vi "InternalStacking.vi"(7 "Cancel Internal Stacking":bool, 10 "Initialize Internal Stacking":bool) -> ()   [LabVIEW 2014]
uses:
  2015 Main Project/InternalStacking.ctl
  2015 Main Project/Robot Global Data.vi
panel:
  in  "Winch Sensor Position":dbl
  out "Winch Cims Setpoint":dbl
  out "Internal Stacking Plate (set)":dbl
  in  "Tote Num Get":dbl
  out "Tote Num Set":dbl
  out "State of Elevator":T1
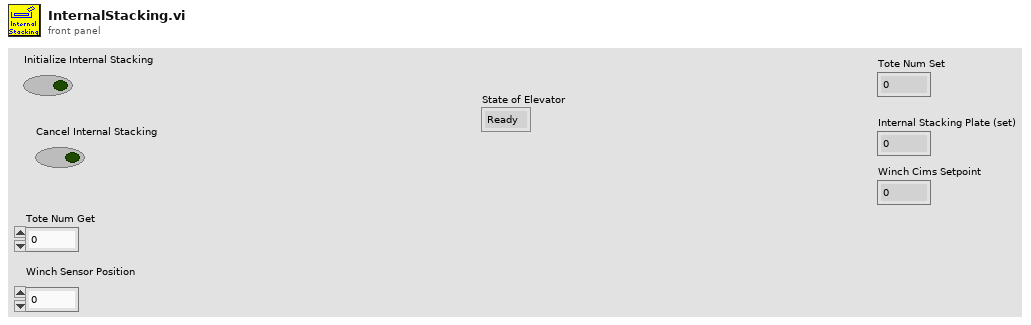
[diagram p1: front panel]
types:
  T1 = typedef "InternalStacking.ctl" = enum16{"Ready", "Extend Plate", "Lift Tote", "Wait For Seated Tote", "Release Tote", "Reset To Bottom Limit ", "Emergency Cancel"}
  T2 = typedef "WPI_ServoDeviceRef.ctl" = cluster{"DeviceStatus":errorcluster, "Controller":T3, "PWM Channel":T4, "DeadBand":T5}
  T3 = typedef "FPGA_TypedefDigitalModule.ctl" = enum16{"Controller 1"}
  T4 = typedef "FPGA_DIOPWMChannel.ctl" = enum8{"PWM 0", "PWM 1", "PWM 2", "PWM 3", "PWM 4", "PWM 5", "PWM 6", "PWM 7", "PWM 8", "PWM 9", "PWM MXP 0", "PWM MXP 1", "PWM MXP 2", "PWM MXP 3", "PWM MXP 4", "PWM MXP 5", "PWM MXP 6", "PWM MXP 7", "PWM MXP 8", "PWM MXP 9", "Invalid"}
  T5 = typedef "WPI_PWMDeadband.ctl" = cluster{"Name":string, "maxPositivePwm":i32, "minPositivePwm":i32, "centerPwm":i32, "maxNegativePwm":i32, "minNegativePwm":i32, "angularRange":u16}
  T6 = typedef "WPI_MotorControlDeviceRef.ctl" = cluster{"DeviceStatus":errorcluster, "Type":T7, "PWM":cluster{"Controller":T3, "PWM Channel":T4, "DeadBand":T5}, "CAN":cluster{"Device Number":u8, "Control Mode":T8, "Semaphore":T9, "Max Vout":dbl, "TalonSRX Control Mode":T10}, "Invert":bool, "TransformRef":T11, "InvTransformRef":T11}
  T7 = typedef "WPI_MotorControlType.ctl" = enum16{"PWM", "CAN", "CANTalonSRX"}
  T8 = typedef "WPI_CANJaguar_ControlMode.ctl" = enum8{"Percent VBus", "Current", "Speed", "Position", "Voltage"}
  T9 = typedef "Semaphore RefNum" = refnum<k1>
  T10 = typedef "WPI_CANTalonSRX_APIControlMode.ctl" = enum8{"Percent VBus", "Speed", "Position", "Slave", "Unchanged / Invalid"}
  T11 = typedef "WPI_PWMTransform_ConPane.ctl" = refnum<vi>
  T12 = typedef "WPI_CANTalonSRX_GlobalStatus.ctl" = cluster{"Applied Throttle":dbl, "Module Enabled":bool, "CAN Error":errorcluster, "Closed Loop Error":dbl, "Forward Limit Switch Closed":bool, "Reverse Limit Switch Closed":bool, "Sensor Position":dbl, "Sensor Velocity":dbl, "Current":dbl, "Sticky Fault - Over Temp":bool, "Sticky Fault - Under Voltage":bool, "Sticky Fault - Forward Limit":bool, "Sticky Fault - Reverse Limit":bool, "Sticky Fault - Forward Soft Limit":bool, "Sticky Fault - Reverse Soft Limit":bool, "Brake is Enabled":bool, "Encoder Position":dbl, "Encoder Velocity":dbl, "Encoder Index Count":dbl, "Encoder A Pin State":bool, "Encoder B Pin State":bool, "Encoder Index Pin State":bool, "Analog In":dbl, "Analog In Velocity":dbl, "Temperature (C)":dbl, "Battery Voltage":dbl}
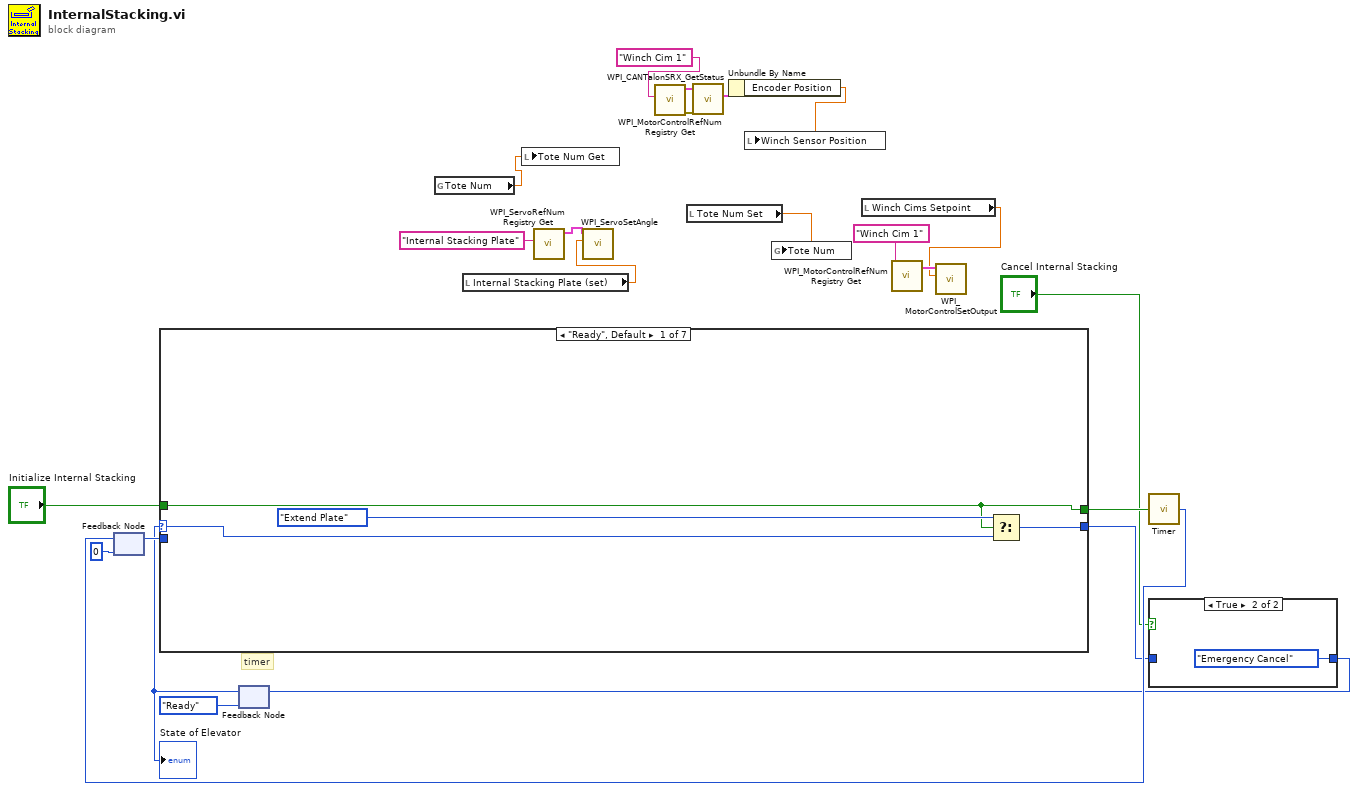
[diagram p0: block diagram]
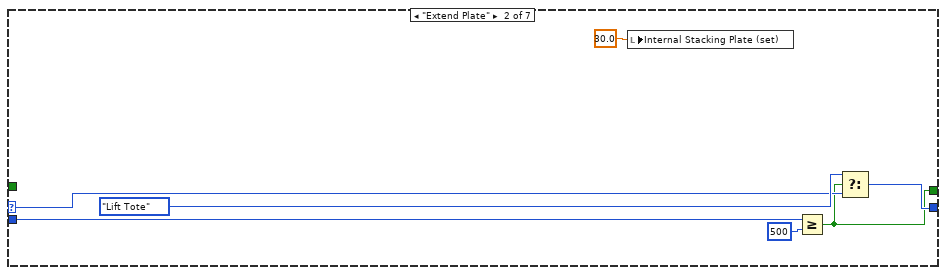
[diagram p3: hidden frame]
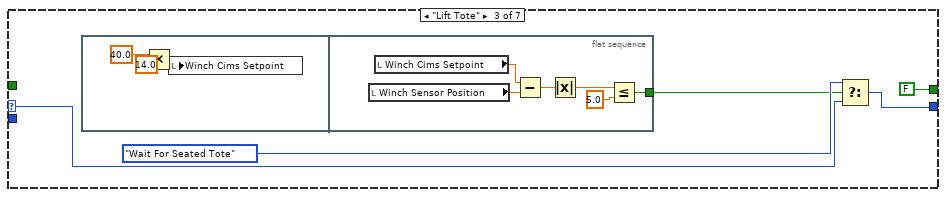
[diagram p4: hidden frame]
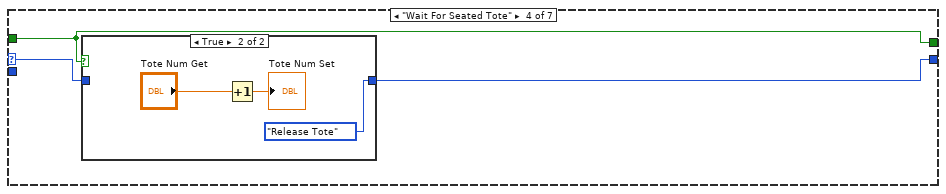
[diagram p5: hidden frame]
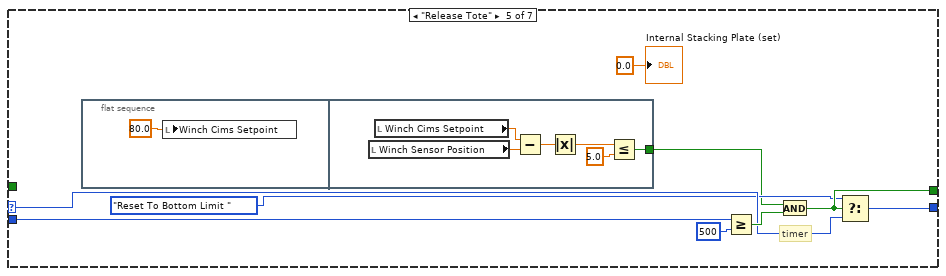
[diagram p7: hidden frame]
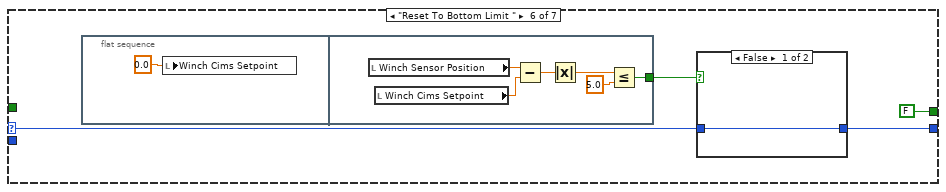
[diagram p8: hidden frame]
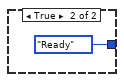
[diagram p9: hidden frame]
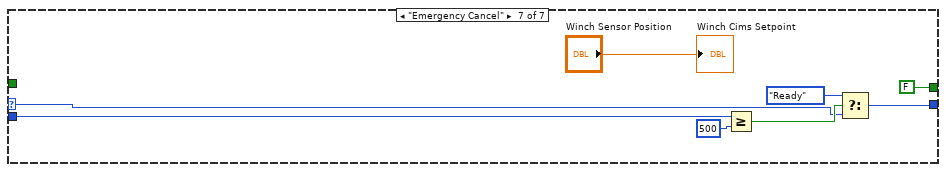
[diagram p10: hidden frame]
diagram:
  # "timer"
  n1 = feedback #1(u64 0 ("Time elapsed")) -> (w20:u64)
  n2 = feedback #2(InternalStacking."Ready" ("State of Elevator")) -> (w14:T1)
  "State of Elevator" <- w14
  n3 = case shown="\"Ready\", Default" w14 {
    selector: w14 -> [w26 w33 w38 w49 w60 w74 w88]
    tunnel: "Initialize Internal Stacking" -> [w24 _ _ w51 _ _ _]
    tunnel: [w25 w32 w37 w50 w58 w75 w87] -> w17
    tunnel: [w24 w29 FALSE ("Initialize Internal Stacking") w51 w61 FALSE ("Initialize Internal Stacking") FALSE] -> w22
    tunnel: w20 -> [_ w31 _ _ w64 _ w86]
    frame "Ready", Default {
      n4 = Select(t=InternalStacking."Extend Plate" ("State of Elevator"), s=w24, f=w26) -> (s? t:f=w25:T1)
    }
    frame "Extend Plate" {
      n5 = local write "Internal Stacking Plate (set)"(30.0 ("Internal Stacking Plate (set)")) -> ()
      n6 = Greater Or Equal?(x=w31, y=500) -> (x >= y?=w29:bool)
      n7 = Select(t=InternalStacking."Lift Tote" ("State of Elevator"), s=w29, f=w33) -> (s? t:f=w32:T1)
    }
    frame "Lift Tote" {
      n8 = flat-sequence {
        tunnel: [w43] -> w36
        frame #0 {
          n9 = Multiply(x=40.0, y=14.0 ("Ejector Motor Set")) -> (x*y=w41:dbl)
          n10 = local write "Winch Cims Setpoint"(w41) -> ()
        }
        frame #1 {
          n11 = local read "Winch Sensor Position"() -> (w48:dbl)
          n12 = local read "Winch Cims Setpoint"() -> (w47:dbl)
          n13 = Subtract(x=w47, y=w48) -> (x-y=w46:dbl)
          n14 = Absolute Value(x=w46) -> (abs(x)=w45:dbl)
          n15 = Less Or Equal?(x=w45, y=5.0) -> (x <= y?=w43:bool)
        }
      }
      n16 = Select(t=InternalStacking."Wait For Seated Tote" ("State of Elevator"), s=w36, f=w38) -> (s? t:f=w37:T1)
    }
    frame "Wait For Seated Tote" {
      n17 = case shown="True" w51 {
        tunnel: [w52 InternalStacking."Release Tote" ("State of Elevator")] -> w50
        tunnel: w49 -> [w52 _]
        frame False {
        }
        frame True {
          n18 = Increment(x="Tote Num Get") -> (x+1=→"Tote Num Set":dbl)
        }
      }
    }
    frame "Release Tote" {
      # "timer"
      n19 = flat-sequence {
        tunnel: [w66] -> w57
        frame #0 {
          n20 = local write "Winch Cims Setpoint"(80.0 ("Ejector Motor Set")) -> ()
        }
        frame #1 {
          n21 = local read "Winch Sensor Position"() -> (w71:dbl)
          n22 = local read "Winch Cims Setpoint"() -> (w70:dbl)
          n23 = Subtract(x=w70, y=w71) -> (x-y=w69:dbl)
          n24 = Absolute Value(x=w69) -> (abs(x)=w68:dbl)
          n25 = Less Or Equal?(x=w68, y=5.0) -> (x <= y?=w66:bool)
        }
      }
      n26 = Greater Or Equal?(x=w64, y=u64 500) -> (x >= y?=w62:bool)
      n27 = And(x=w57, y=w62) -> (x .and. y?=w61:bool)
      n28 = Select(t=InternalStacking."Reset To Bottom Limit " ("State of Elevator"), s=w61, f=w60) -> (s? t:f=w58:T1)
      "Internal Stacking Plate (set)" <- 0.0 ("Internal Stacking Plate (set)")
    }
    frame "Reset To Bottom Limit " {
      n29 = flat-sequence {
        tunnel: [w77] -> w73
        frame #0 {
          n30 = local write "Winch Cims Setpoint"(0.0 ("Ejector Motor Set")) -> ()
        }
        frame #1 {
          n31 = local read "Winch Sensor Position"() -> (w81:dbl)
          n32 = local read "Winch Cims Setpoint"() -> (w82:dbl)
          n33 = Subtract(x=w81, y=w82) -> (x-y=w80:dbl)
          n34 = Absolute Value(x=w80) -> (abs(x)=w79:dbl)
          n35 = Less Or Equal?(x=w79, y=5.0) -> (x <= y?=w77:bool)
        }
      }
      n36 = case shown="False" w73 {
        tunnel: [w83 InternalStacking."Ready" ("State of Elevator")] -> w75
        tunnel: w74 -> [w83 _]
        frame False {
        }
        frame True {
        }
      }
    }
    frame "Emergency Cancel" {
      n37 = Greater Or Equal?(x=w86, y=u64 500) -> (x >= y?=w90:bool)
      n38 = Select(t=InternalStacking."Ready" ("State of Elevator"), s=w90, f=w88) -> (s? t:f=w87:T1)
      "Winch Cims Setpoint" <- "Winch Sensor Position"
    }
  }
  n39 = global read "Robot Global Data.vi" "Tote Num"() -> (w13:dbl)
  n40 = local read "Internal Stacking Plate (set)"() -> (w10:dbl)
  n41 = local write "Tote Num Get"(w13) -> ()
  n42 = call <vilib>:"WPI_ServoRefNum Registry Get.vi"("refnum name"="Internal Stacking Plate") -> ("ServoDeviceRef"=w9:T2)  [unwired: 9 in, 1 out]
  n43 = call <vilib>:"WPI_ServoSetAngle.vi"("Angle"=w10, "ServoDeviceRef"=w9) -> ()  [unwired: 8 in, 2 out]
  n44 = call <vilib>:"WPI_MotorControlRefNum Registry Get.vi"("refnum name"="Winch Cim 1") -> ("error out"=w6:errorcluster, "MotorControlDevRef"=w7:T6)  [unwired: 9 in]
  n45 = local read "Tote Num Set"() -> (w12:dbl)
  n46 = call <vilib>:"WPI_CANTalonSRX_GetStatus.vi"("error in (no error)"=w6, "CAN Talon SRX Ref"=w7) -> ("Talon SRX Status"=w8:T12)  [unwired: 7 in, 2 out]
  n47 = Unbundle By Name(w8) -> ("Encoder Position"=w5:dbl)
  n48 = local write "Winch Sensor Position"(w5) -> ()
  n49 = global write "Robot Global Data.vi" "Tote Num"(w12) -> ()
  n50 = local read "Winch Cims Setpoint"() -> (w2:dbl)
  n51 = call <vilib>:"WPI_MotorControlRefNum Registry Get.vi"("refnum name"="Winch Cim 1") -> ("MotorControlDevRef"=w3:T6)  [unwired: 9 in, 1 out]
  n52 = call <vilib>:"WPI_MotorControlSetOutput.vi"("Output"=w2, "MotorControlDevRef"=w3) -> ()  [unwired: 7 in, 3 out]
  n53 = call "Timer.vi"("Set Timer"=w22) -> ("Time elapsed"=w21:u64)
  n54 = feedback-in #1(w21) -> ()
  n55 = case shown="True" "Cancel Internal Stacking" {
    tunnel: [w93 InternalStacking."Emergency Cancel" ("State of Elevator")] -> w16
    tunnel: w17 -> [w93 _]
    frame False {
    }
    frame True {
    }
  }
  n56 = feedback-in #2(w16) -> ()
